vi "Init_Pruefung_Oben.vi"(8 "Fehler in":errorcluster, 11 "Cluster in":T1) -> (0 "Fehler out":errorcluster, 3 "Cluster out":T1)   [LabVIEW 2024]
doc: "Schreibt den Speicherpfad für die Bilder in das Cluster und inkrementiert die Kontaktnummer."
uses:
  Typdefinitionen/Cluster.ctl
  <vilib>/userDefined/High Color/IMAQdx.ctl
  <vilib>/DATA AHEAD/SP7/typedefs/S7 Connection.ctl
  <vilib>/DATA AHEAD/SP7/typedefs/PLC Type.ctl
  <vilib>/vision/Image Controls.llb/IMAQ Image.ctl
  Typdefinitionen/Koordinatensystem.ctl
  Typdefinitionen/Statistik.ctl
  <vilib>/Utility/file.llb/Read Delimited Spreadsheet (DBL).vi
  Globale Variablen.vi
  <vilib>/DATA AHEAD/SP7/SP7.lvlib
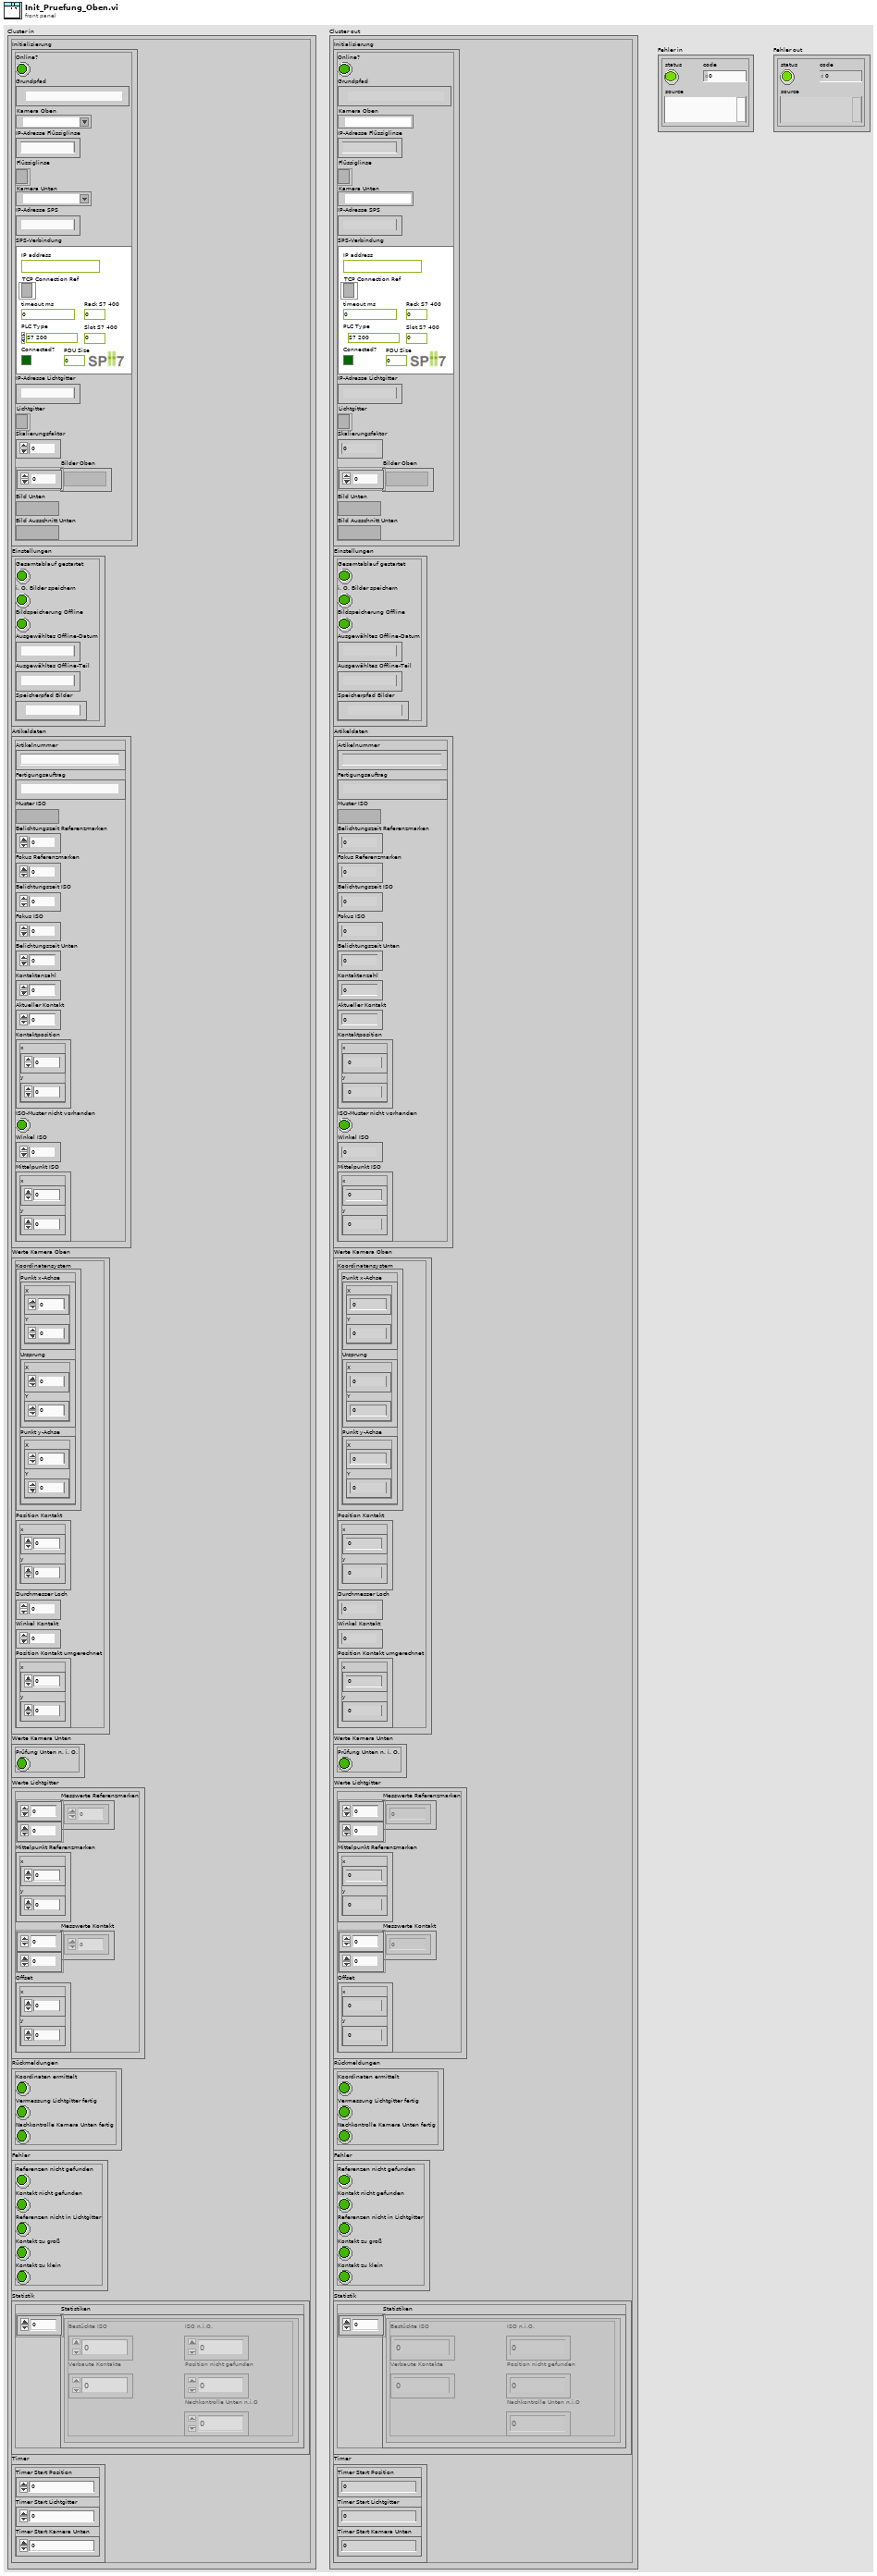
[diagram p1: front panel]
types:
  T1 = typedef "Cluster.ctl" = cluster{"Initialisierung":cluster{"Online?":bool, "Grundpfad":path, "Kamera Oben":T2, "IP-Adresse Flüssiglinse":string, "Flüssiglinse":refnum<k5>, "Kamera Unten":T2, "IP-Adresse SPS":string, "SPS-Verbindung":T3, "IP-Adresse Lichtgitter":string, "Lichtgitter":refnum<k5>, "Skalierungsfaktor":dbl, "Bilder Oben":T6[], "Bild Unten":T6, "Bild Ausschnitt Unten":T6}, "Einstellungen":cluster{"Gesamtablauf gestartet":bool, "i. O. Bilder speichern":bool, "Bildspeicherung Offline":bool, "Ausgewähltes Offline-Datum":string, "Ausgewähltes Offline-Teil":string, "Speicherpfad Bilder":path}, "Artikeldaten":cluster{"Artikelnummer":string, "Fertigungsauftrag":string, "Muster ISO":T6, "Belichtungszeit Referenzmarken":dbl, "Fokus Referenzmarken":dbl, "Belichtungszeit ISO":dbl, "Fokus ISO":dbl, "Belichtungszeit Unten":dbl, "Kontaktanzahl":u32, "Aktueller Kontakt":i16, "Kontaktposition":cluster{"x":sgl, "y":sgl}, "ISO-Muster nicht vorhanden":bool, "Winkel ISO":sgl, "Mittelpunkt ISO":cluster{"x":dbl, "y":dbl}}, "Werte Kamera Oben":cluster{"Koordinatensystem":T7, "Position Kontakt":cluster{"x":dbl, "y":dbl}, "Durchmesser Loch":dbl, "Winkel Kontakt":dbl, "Position Kontakt umgerechnet":cluster{"x":dbl, "y":dbl}}, "Werte Kamera Unten":cluster{"Prüfung Unten n. i. O.":bool}, "Werte Lichtgitter":cluster{"Messwerte Referenzmarken":dbl[][], "Mittelpunkt Referenzmarken":cluster{"x":dbl, "y":dbl}, "Messwerte Kontakt":dbl[][], "Offset":cluster{"x":dbl, "y":dbl}}, "Rückmeldungen":cluster{"Koordinaten ermittelt":bool, "Vermessung Lichtgitter fertig":bool, "Nachkontrolle Kamera Unten fertig":bool}, "Fehler":cluster{"Referenzen nicht gefunden":bool, "Kontakt nicht gefunden":bool, "Referenzen nicht in Lichtgitter":bool, "Kontakt zu groß":bool, "Kontakt zu klein":bool}, "Statistik":cluster{"Statistiken":T8[]}, "Timer":cluster{"Timer Start Position":u32, "Timer Start Lichtgitter":u32, "Timer Start Kamera Unten":u32}}
  T2 = typedef "IMAQdx.ctl" = refnum<k21>
  T3 = typedef "SP7.lvlib/S7 Connection.ctl" = cluster{"TCP Connection Ref":refnum<k5>, "IP address":string, "timeout ms":i32, "Connected?":bool, "PLC Type":T4, "Rack S7 400":u8, "Slot S7 400":u8, "PDU Size":u16, "connection semaphore":T5}
  T4 = typedef "SP7.lvlib/PLC Type.ctl" = enum16{"S7 200", "S7 300/400", "S7 1200", "S7 1500", "LOGO!8"}
  T5 = typedef "Semaphore RefNum" = refnum<k1>
  T6 = typedef "IMAQ Image.ctl" = refnum<image>
  T7 = typedef "Koordinatensystem.ctl" = cluster{"Punkt x-Achse":cluster{"X":sgl, "Y":sgl}, "Ursprung":cluster{"X":sgl, "Y":sgl}, "Punkt y-Achse":cluster{"X":sgl, "Y":sgl}}
  T8 = typedef "Statistik.ctl" = cluster{"Bestückte ISO":u32, "Verbaute Kontakte":u32, "ISO n.i.O.":u32, "Nachkontrolle Unten n.i.O":u32, "Position nicht gefunden":u32}
  T9 = cluster{"Koordinatensystem":T7, "Position Kontakt":cluster{"x":dbl, "y":dbl}, "Durchmesser Loch":dbl, "Winkel Kontakt":dbl, "Position Kontakt umgerechnet":cluster{"x":dbl, "y":dbl}}
  T10 = cluster{"Koordinaten ermittelt":bool, "Vermessung Lichtgitter fertig":bool, "Nachkontrolle Kamera Unten fertig":bool}
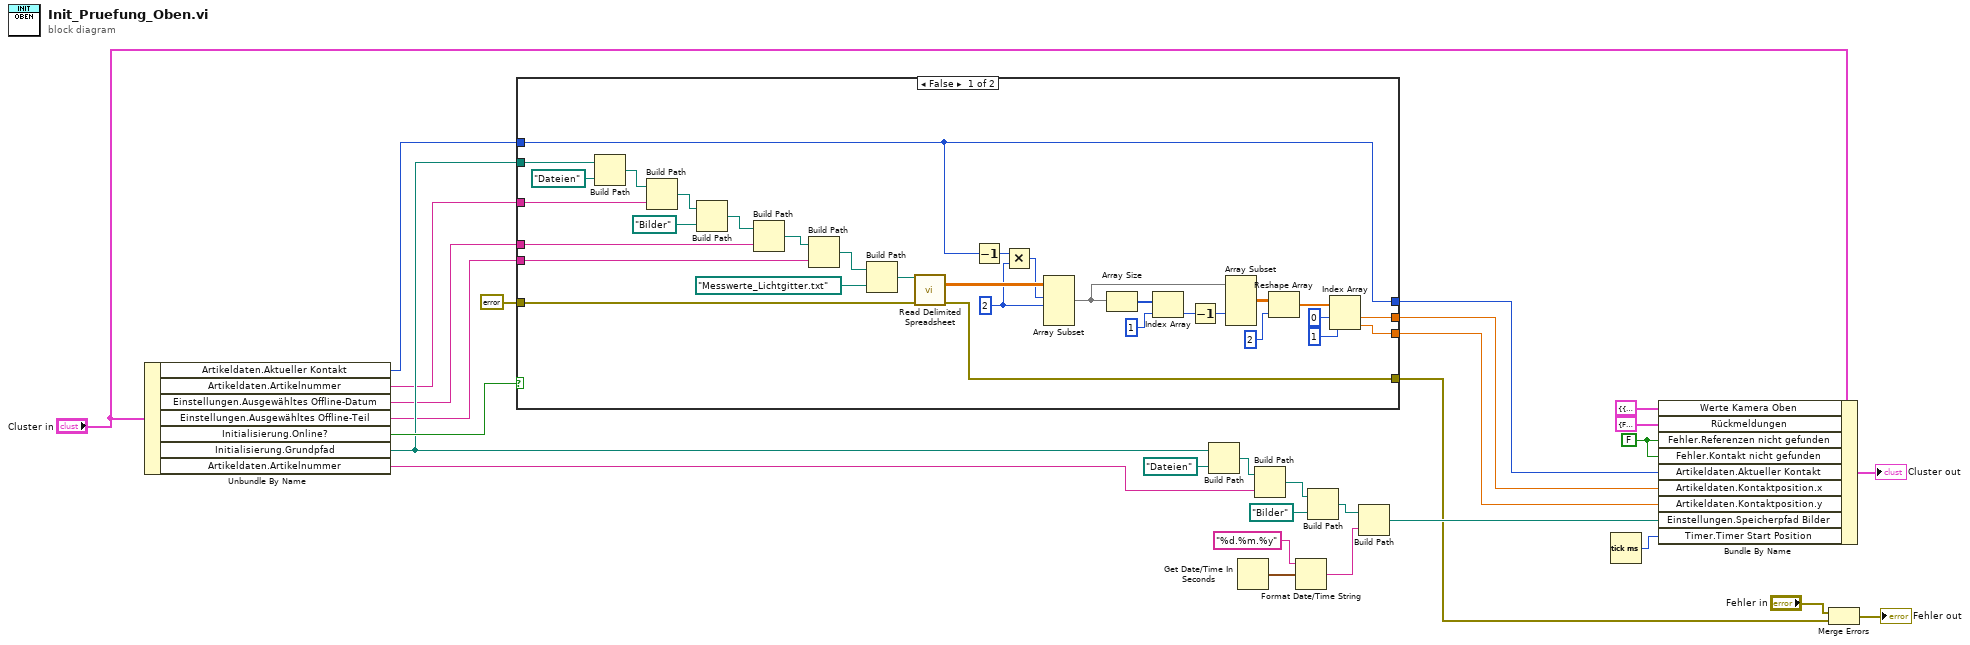
[diagram p0: block diagram]
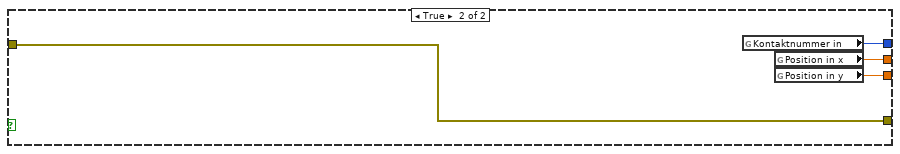
[diagram p2: hidden frame]
diagram:
  w2 = FALSE ("Fehler.Referenzen nicht gefunden")
  n1 = Unbundle By Name("Cluster in") -> ("Artikeldaten.Aktueller Kontakt"=w12:i16, "Artikeldaten.Artikelnummer"=w15:string, "Einstellungen.Ausgewähltes Offline-Datum"=w14:string, "Einstellungen.Ausgewähltes Offline-Teil"=w13:string, "Initialisierung.Online?"=w17:bool, "Initialisierung.Grundpfad"=w16:path, "Artikeldaten.Artikelnummer"=w28:string)
  n2 = case shown="False" w17 {
    tunnel: w16 -> [w45 _]
    tunnel: w15 -> [w44 _]
    tunnel: w14 -> [w43 _]
    tunnel: w13 -> [w42 _]
    tunnel: w12 -> [w32 _]
    tunnel: [w34 w64] -> w10
    tunnel: [w33 w65] -> w11
    tunnel: [w32 w63] -> w9
    tunnel: errorcluster {"status"=FALSE, "code"=0, "source"=""} ("error in (no error)") -> [w31 w62]
    tunnel: [w30 w62] -> w4
    frame False {
      w47 = 2 ("length")
      n3 = Build Path(base path=w45, name or relative path=path "Dateien") -> (appended path=w58:path)
      n4 = Build Path(base path=w58, name or relative path=w44) -> (appended path=w51:path)
      n5 = Build Path(base path=w51, name or relative path=path "Bilder") -> (appended path=w57:path)
      n6 = Build Path(base path=w57, name or relative path=w43) -> (appended path=w52:path)
      n7 = Build Path(base path=w52, name or relative path=w42) -> (appended path=w53:path)
      n8 = Build Path(base path=w53, name or relative path=path "Messwerte_Lichtgitter.txt") -> (appended path=w54:path)
      n9 = call-poly <vilib>:"Read Delimited Spreadsheet.vi"("file path (dialog if empty)"=w54, "error in (no error)"=w31) -> ("all rows"=w61:dbl[][], "error out"=w30:errorcluster)  [unwired: 8 in, 4 out]
      n10 = Decrement(x=w32) -> (x-1=w55:i16)
      n11 = Multiply(x=w55, y=w47) -> (x*y=w56:i32)
      n12 = Array Subset(array=w61, index (row)=w56, length (row)=w47) -> (w60:dbl[][])  [unwired: 2 in]
      n13 = Array Size(array=w60) -> (size(s)=w59:i32[])
      n14 = Index Array(array=w59, index=1) -> (element=w41:i32)
      n15 = Decrement(x=w41) -> (x-1=w40:i32)
      n16 = Array Subset(array=w60, index (col)=w40) -> (w39:dbl[][])  [unwired: 3 in]
      n17 = Reshape Array(w39, 2 ("dimension size")) -> (w37:dbl[])
      n18 = Index Array(array=w37, index #1=0 ("index"), index #2=1 ("index")) -> (element #1=w34:dbl, element #2=w33:dbl)
    }
    frame True {
      n19 = global read "Globale Variablen.vi" "Kontaktnummer in"() -> (w63:i16)
      n20 = global read "Globale Variablen.vi" "Position in x"() -> (w64:sgl)
      n21 = global read "Globale Variablen.vi" "Position in y"() -> (w65:sgl)
    }
  }
  n22 = Build Path(base path=w16, name or relative path=path "Dateien") -> (appended path=w22:path)
  n23 = Get Date/Time In Seconds() -> (seconds since 1Jan1904=w26:timestamp)
  n24 = Build Path(base path=w22, name or relative path=w28) -> (appended path=w21:path)
  n25 = Format Date/Time String(time format string (%c)="%d.%m.%y", seconds (now)=w26) -> (date/time string=w25:string)  [unwired: 1 in]
  n26 = Build Path(base path=w21, name or relative path=path "Bilder") -> (appended path=w20:path)
  n27 = Build Path(base path=w20, name or relative path=w25) -> (appended path=w18:path)
  n28 = Tick Count (ms)() -> (millisecond timer value=w3:u32)
  n29 = Bundle By Name(cluster="Cluster in", "Werte Kamera Oben"=T9 {"Koordinatensystem"={"Punkt x-Achse"={"X"=0.0, "Y"=0.0}, "Ursprung"={"X"=0.0, "Y"=0.0}, "Punkt y-Achse"={"X"=0.0, "Y"=0.0}}, "Position Kontakt"={"x"=0.0, "y"=0.0}, "Durchmesser Loch"=0.0, "Winkel Kontakt"=0.0, "Position Kontakt umgerechnet"={"x"=0.0, "y"=0.0}}, "Rückmeldungen"=T10 {"Koordinaten ermittelt"=FALSE, "Vermessung Lichtgitter fertig"=FALSE, "Nachkontrolle Kamera Unten fertig"=FALSE}, "Fehler.Referenzen nicht gefunden"=w2, "Fehler.Kontakt nicht gefunden"=w2, "Artikeldaten.Aktueller Kontakt"=w9, "Artikeldaten.Kontaktposition.x"=w10, "Artikeldaten.Kontaktposition.y"=w11, "Einstellungen.Speicherpfad Bilder"=w18, "Timer.Timer Start Position"=w3) -> (→"Cluster out":T1)
  n30 = Merge Errors("Fehler in", w4) -> (→"Fehler out":errorcluster)
